vi "Autonomous Independent.vi"() -> ()   [LabVIEW 2017]
doc: "This VI is called when autonomous begins, and will automatically be terminated when autonomous ends. You can carry out timed or sensor driven robot movement independently without needing to return to the caller."
uses:
  <vilib>/Rock Robotics/WPI/Utilities/WPI_GetSetVariantRefNum.vi
panel:
  in  "Distance":dbl
  out "Angle":dbl
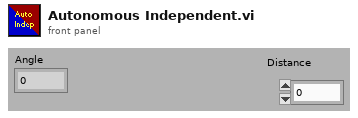
[diagram p1: front panel]
types:
  T1 = typedef "WPI_EncoderDevRef.ctl" = cluster{"DevStatus":errorcluster, "EncoderIndex":T2, "CounterIndex":T3, "DistancePerCount":dbl, "Decoding Type":T4}
  T2 = typedef "FPGA_EncoderIdx.ctl" = enum8{"Enc 0", "Enc 1", "Enc 2", "Enc 3", "Enc 4", "Enc 5", "Enc 6", "Enc 7", "Invalid"}
  T3 = typedef "FPGA_CounterCtrSystemIndex.ctl" = enum8{"Ctr 0", "Ctr 1", "Ctr 2", "Ctr 3", "Ctr 4", "Ctr 5", "Ctr 6", "Ctr 7", "Invalid"}
  T4 = typedef "WPI_EncoderType.ctl" = enum16{"1x", "2x", "4x"}
  T5 = typedef "WPI_RobotDriveDevRef.ctl" = cluster{"DevStatus":errorcluster, "Motors[]":T6[], "Square Inputs":bool, "Max Output":dbl}
  T6 = typedef "WPI_MotorControlDeviceRef.ctl" = cluster{"DeviceStatus":errorcluster, "Type":T7, "PWM":cluster{"PWM Channel":T8, "DeadBand":T9}, "CAN":cluster{"Device Number":u8, "SetOutput VI Ref":variant, "GetOutput VI Ref":variant, "Enable VI Ref":variant, "Disable VI Ref":variant, "Data":variant}, "Invert":bool, "DIO PWM":cluster{"PWM \"Enable\" Channel":T8, "DIOChannel":T10, "PWM Rate":dbl}}
  T7 = typedef "WPI_MotorControlType.ctl" = enum16{"PWM", "CAN", "DIO PWM"}
  T8 = typedef "FPGA_DIOPWMChannel.ctl" = enum8{"PWM 0", "PWM 1", "PWM 2", "PWM 3", "PWM 4", "PWM 5", "PWM 6", "PWM 7", "PWM 8", "PWM 9", "PWM MXP 0", "PWM MXP 1", "PWM MXP 2", "PWM MXP 3", "PWM MXP 4", "PWM MXP 5", "PWM MXP 6", "PWM MXP 7", "PWM MXP 8", "PWM MXP 9", "Invalid"}
  T9 = typedef "WPI_PWMDeadband.ctl" = cluster{"Name":string, "maxPositivePwm":i32, "minPositivePwm":i32, "centerPwm":i32, "maxNegativePwm":i32, "minNegativePwm":i32, "angularRange":u16}
  T10 = typedef "FPGA_DIOChannel.ctl" = enum8{"DIO 0", "DIO 1", "DIO 2", "DIO 3", "DIO 4", "DIO 5", "DIO 6", "DIO 7", "DIO 8", "DIO 9", "DIO MXP 0", "DIO MXP 1", "DIO MXP 2", "DIO MXP 3", "DIO MXP 4", "DIO MXP 5", "DIO MXP 6", "DIO MXP 7", "DIO MXP 8", "DIO MXP 9", "DIO MXP 10", "DIO MXP 11", "DIO MXP 12", "DIO MXP 13", "DIO MXP 14", "DIO MXP 15", "SPI Port CS1", "SPI Port CS2", "SPI Port CS3", "SPI Port MISO", "SPI Port MOSI", "Invalid"}
  T11 = typedef "WPI_GyroDevRef.ctl" = cluster{"DevStatus":errorcluster, "Analog Channel":T12, "Gain (VoltsPerDegree/Second)":dbl, "Gyro Type":enum16{"Analog", "XRS450"}, "Handle":i32, "SPI Bus":T13, "Device Found":bool, "Sample Rate":dbl, "Calibrate On Open":bool, "Offset":dbl}
  T12 = typedef "FPGA_AIChannel.ctl" = enum8{"AI 0", "AI 1", "AI 2", "AI 3", "AI MXP 0", "AI MXP 1", "AI MXP 2", "AI MXP 3", "Invalid"}
  T13 = typedef "spi_bus.ctl" = enum16{"SPI On-Board, CS0", "SPI On-Board, CS1", "SPI On-Board, CS2", "SPI On-Board, CS3", "SPI MXP", "Invalid"}
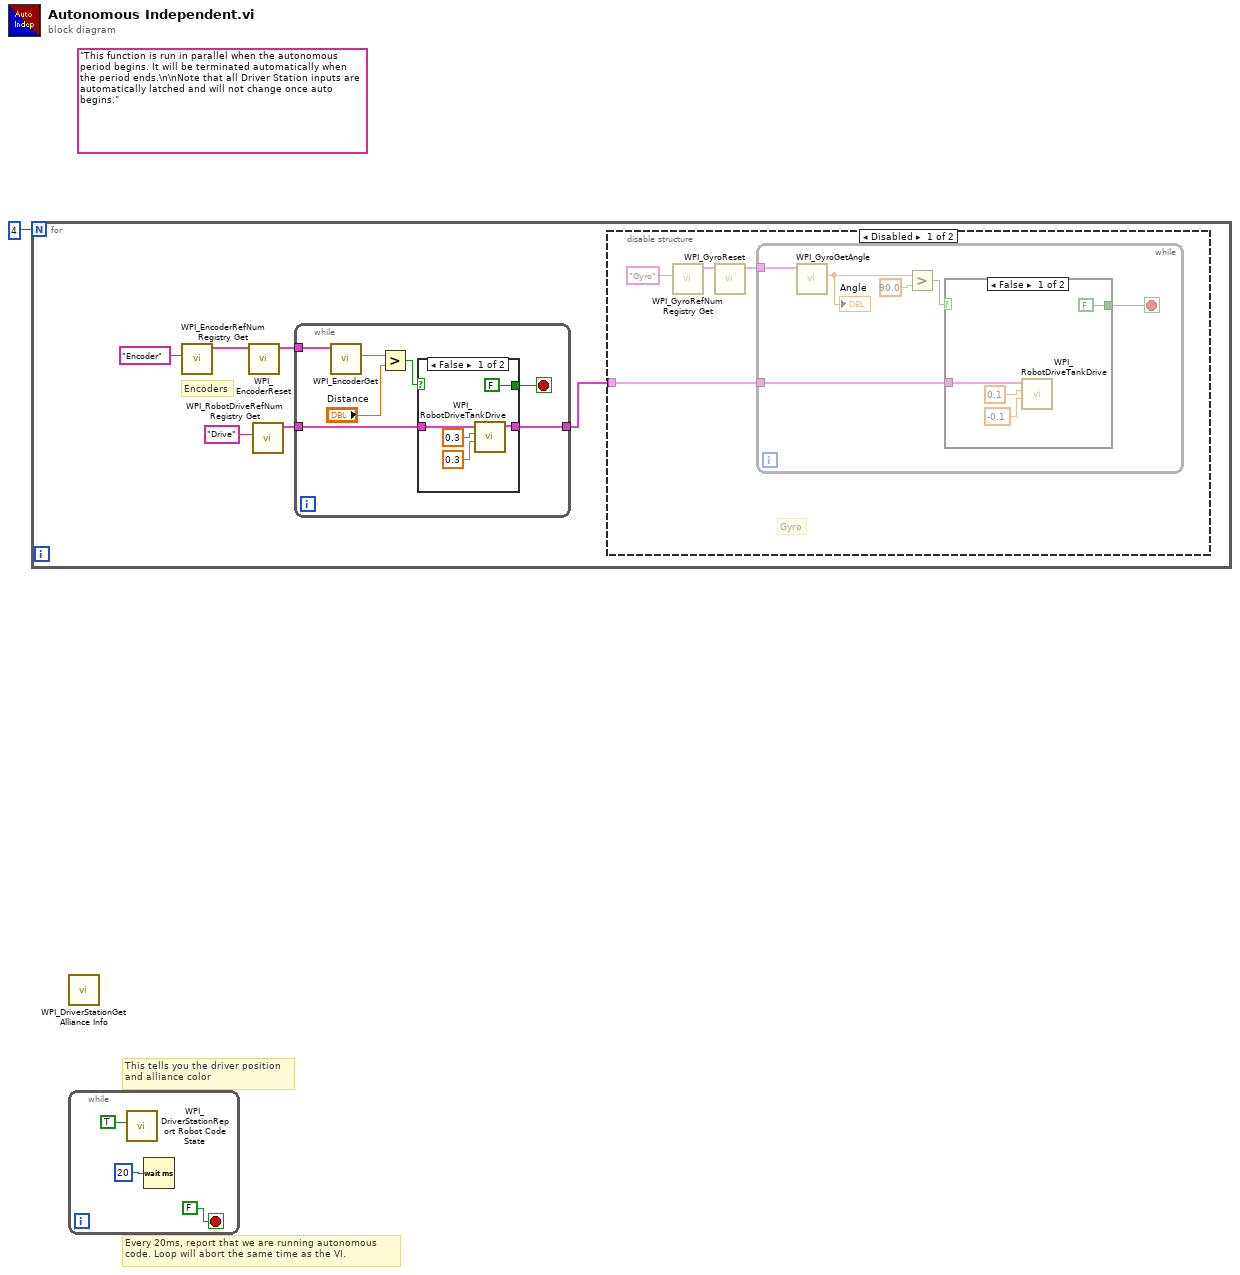
[diagram p0: block diagram]
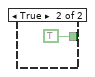
[diagram p2: hidden frame]
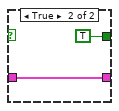
[diagram p4: hidden frame]
diagram:
  (unwired) "This function is run in parallel when the autonomous period begins. It will be terminated automatically when the period ends.\n\nNote that all Driver Station inputs are automatically latched and will not change once auto begins."
  # "Every 20ms, report that we are running autonomous\ncode. Loop will abort the same time as the VI."
  # "This tells you the driver position\nand alliance color"
  n1 = for {
    N: 4 -> [_]
    # "Encoders"
    n2 = call <vilib>:"WPI_EncoderRefNum Registry Get.vi"("refnum name"="Encoder") -> ("EncoderDevRef"=w5:T1)  [unwired: 9 in, 1 out]
    n3 = call <vilib>:"WPI_EncoderReset.vi"("EncoderDevRef"=w5) -> ("EncoderDevRef"=w7:T1)  [unwired: 9 in, 1 out]
    n4 = call <vilib>:"WPI_RobotDriveRefNum Registry Get.vi"("refnum name"="Drive") -> ("RobotDriveDevRef"=w2:T5)  [unwired: 9 in, 1 out]
    n5 = while {
      tunnel: w7 -> [w29]
      tunnel: [w27] -> w6
      tunnel: w2 -> [w23]
      stop <- w28 stop-if-true
      n6 = call <vilib>:"WPI_EncoderGet.vi"("EncoderDevRef"=w29) -> ("Distance"=w25:dbl)  [unwired: 5 in, 5 out]
      n7 = Greater?(x=w25, y="Distance") -> (0:w26:bool)
      n8 = case shown="False" w26 {
        tunnel: [FALSE TRUE] -> w28
        tunnel: [w30 w35] -> w27
        tunnel: w23 -> [w31 w35]
        frame False {
          n9 = call <vilib>:"WPI_RobotDriveTankDrive.vi"("Right axis value"=0.3, "Left axis value"=0.3, "RobotDriveDevRef"=w31) -> ("RobotDriveDevRef"=w30:T5)  [unwired: 6 in, 2 out]
        }
        frame True {
        }
      }
    }
    n10 = disable-structure shown="Disabled" {
      disable-tunnel: w6 -> [w11 _]
      frame Disabled {
        # "Gyro"
        n11 = call <vilib>:"WPI_GyroRefNum Registry Get.vi"("refnum name"="Gyro") -> ("GyroDevRef"=w10:T11)  [unwired: 9 in, 1 out]
        n12 = call <vilib>:"WPI_GyroReset.vi"("GyroDevRef"=w10) -> ("GyroDevRef"=w9:T11)  [unwired: 9 in, 1 out]
        n13 = while {
          tunnel: w11 -> [w13]
          tunnel: w9 -> [w12]
          stop <- w14 stop-if-true
          n14 = call <vilib>:"WPI_GyroGetAngle.vi"("GyroDevRef"=w12) -> ("Angle"=w17:dbl)  [unwired: 6 in, 4 out]
          "Angle" <- w17
          n15 = Greater?(x=w17, y=90.0) -> (0:w15:bool)
          n16 = case shown="False" w15 {
            tunnel: [FALSE TRUE] -> w14
            tunnel: w13 -> [w20 _]
            frame False {
              n17 = call <vilib>:"WPI_RobotDriveTankDrive.vi"("Right axis value"=-0.1, "Left axis value"=0.1, "RobotDriveDevRef"=w20) -> ()  [unwired: 6 in, 3 out]
            }
            frame True {
            }
          }
        }
      }
      frame Enabled {
      }
    }
  }
  n18 = call <vilib>:"WPI_DriverStationGet Alliance Info.vi"() -> ()  [unwired: 12 out]
  n19 = while {
    stop <- FALSE stop-if-true
    n20 = call <vilib>:"WPI_DriverStationReport Robot Code State.vi"("Autonomous"=TRUE) -> ()  [unwired: 10 in, 1 out]
    n21 = Wait (ms)(milliseconds to wait=u32 20) -> ()  [unwired: 1 out]
  }
